vi "System@Delay__Parameter.vi"(1 "ParamterIn":string) -> (0 "ParamterOut":string)   [LabVIEW 2020]
panel:
  in  "Second":string(combo)
  in  "Confirm":bool
  # "System@Delay $Second"
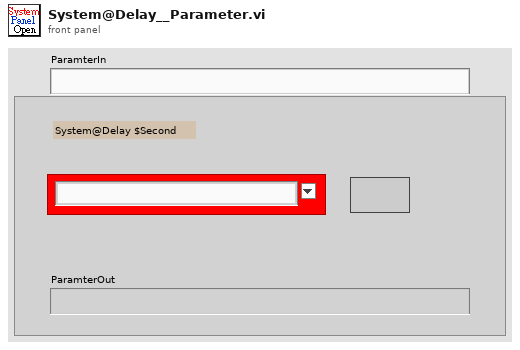
[diagram p1: front panel]
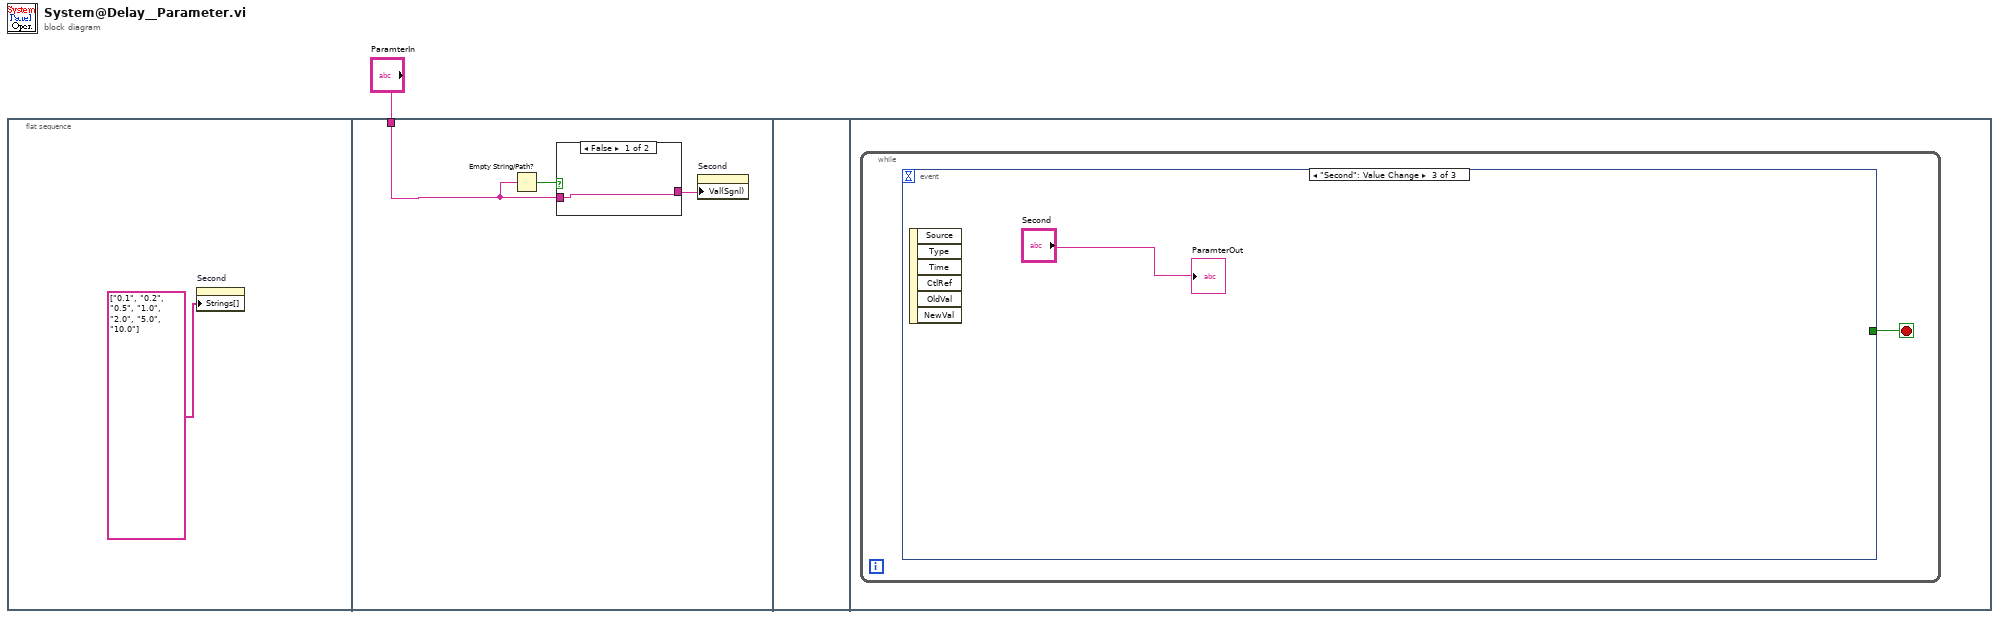
[diagram p0: block diagram]
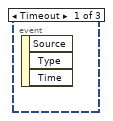
[diagram p3: hidden frame]
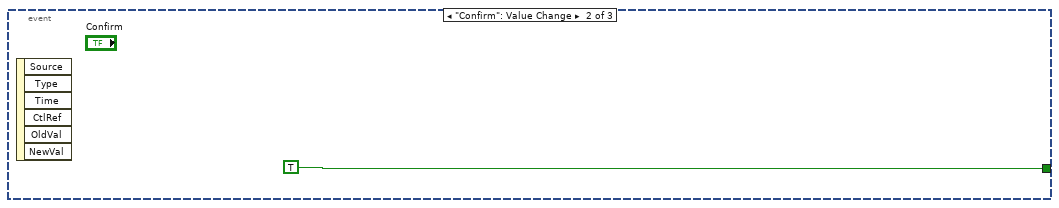
[diagram p4: hidden frame]
diagram:
  n1 = flat-sequence {
    tunnel: "ParamterIn" -> [w3]
    frame #0 {
      n2 = property on="Second" class="CmbBox"("Strings[]"=string[] ["0.1", "0.2", "0.5", "1.0", "2.0", "5.0", "10.0"] ("Strings []")) -> ()  [unwired: 2 in, 2 out]
    }
    frame #1 {
      n3 = Empty String/Path?(string/path=w3) -> (empty?=w5:bool)
      n4 = case shown="False" w5 {
        tunnel: w3 -> [w6 w7]
        tunnel: [w6 w7] -> w4
        frame False {
        }
        frame True {
        }
      }
      n5 = property on="Second" class="CmbBox"("Val(Sgnl)"=w4) -> ()  [unwired: 2 in, 2 out]
    }
    frame #2 {
    }
    frame #3 {
      n6 = while {
        stop <- w8 stop-if-true
        n7 = event shown="[2] \"Second\": Value Change" {
          selector: _ -> [_ _ _]
          dyn-events: _ -> [_ _ _]
          timeout: _ -> [_ _ _]
          tunnel: [_ TRUE _] -> w8
          event Timeout {
            n8 = event-data() -> ()  [unwired: 1 in, 3 out]
          }
          event "Confirm": Value Change {
            n9 = event-data() -> ()  [unwired: 1 in, 6 out]
          }
          event "Second": Value Change {
            n10 = event-data() -> ()  [unwired: 1 in, 6 out]
            "ParamterOut" <- "Second"
          }
        }
      }
    }
  }
